vi "Thermocouple (SubVI).vi"(10 "Boolean":bool, 11 "mean":dbl) -> (3 "T":dbl)   [LabVIEW 2023]
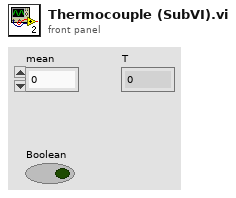
[diagram p1: front panel]
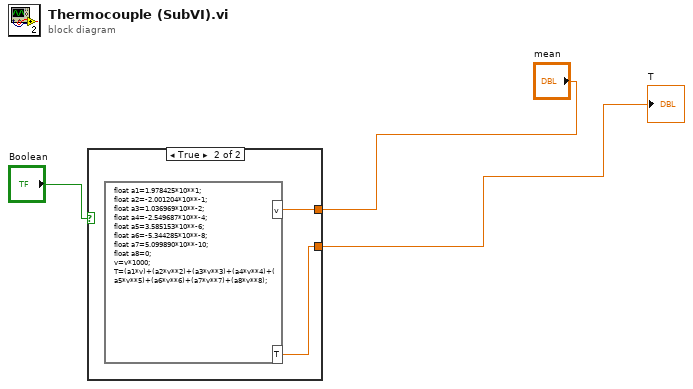
[diagram p0: block diagram]
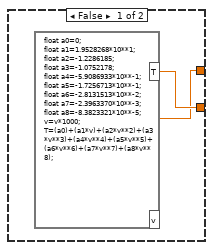
[diagram p2: hidden frame]
diagram:
  n1 = case shown="True" "Boolean" {
    tunnel: [w5 w6] -> w3
    tunnel: "mean" -> [w4 w7]
    frame False {
      n2 = formula code="float a0=0;\nfloat a1=1.9528268*10**1;\nfloat a2=-1.2286185;\nfloat a3=-1.0752178;\nfloat a4=-5.9086933*10**-1;\nfloat a5=-1.7256713*10**-1;\nfloat a6=-2.8131513*10**-2;\nfloat a7=-2.3963370*10**-3;\nfloat a8=-8.3823321*10**-5;\nv=v*1000;\nT=(a0)+(a1*v)+(a2*v**2)+(a3*v**3)+(a4*v**4)+(a5*v**5)+(a6*v**6)+(a7*v**7)+(a8*v**8);"("v"=w4) -> ("T"=w5:dbl)
    }
    frame True {
      n3 = formula code="float a1=1.978425*10**1;\nfloat a2=-2.001204*10**-1;\nfloat a3=1.036969*10**-2;\nfloat a4=-2.549687*10**-4;\nfloat a5=3.585153*10**-6;\nfloat a6=-5.344285*10**-8;\nfloat a7=5.099890*10**-10;\nfloat a8=0;\nv=v*1000;\nT=(a1*v)+(a2*v**2)+(a3*v**3)+(a4*v**4)+(a5*v**5)+(a6*v**6)+(a7*v**7)+(a8*v**8);"("v"=w7) -> ("T"=w6:dbl)
    }
  }
  "T" <- w3
